vi "Recieve M1M3 State Event.vi"(8 "error in (no error)":errorcluster, 11 "M1M3 Support Events in":refnum<class "M1M3 Support Events.lvclass">) -> (0 "error out":errorcluster, 2 "M1M3 State":string, 3 "M1M3 Support Events out":refnum<class "M1M3 Support Events.lvclass">)   [LabVIEW 2016, in "M1M3 Support Events.lvclass"]
uses:
  M1M3 Support Events.lvclass
  M1M3 Support Events.lvclass/M1M3 Support Events.ctl
  Typedefs/StateTypes.ctl
  Typedefs/M1M3SupportEUI_TypeDefs.lvlib
  View/M1M3SupportEUI_Views.lvlib
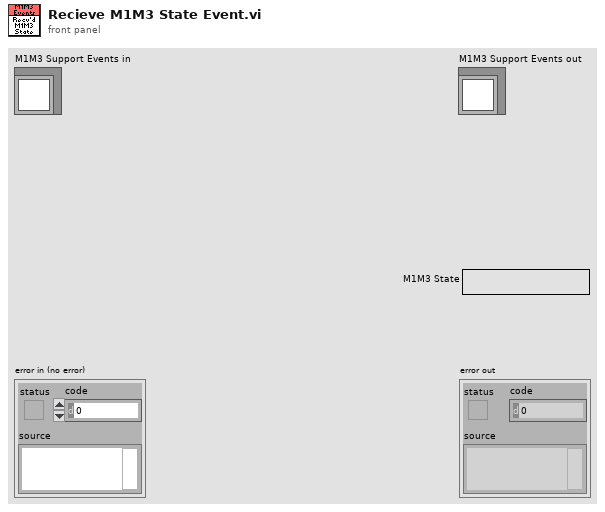
[diagram p1: front panel]
types:
  T1 = typedef "M1M3SupportEUI_TypeDefs.lvlib/M1M3 Support Events.ctl" = cluster{"M1M3 Support State":refnum<user-event>, "Inclinometer  Data":refnum<user-event>, "IMS Data":refnum<user-event>, "FA Status":refnum<user-event>, "SAL Connected":refnum<user-event>, "HP Data":refnum<user-event>, "HP Status":refnum<user-event>, "Accelerometer Data":refnum<user-event>, "FPGA Data":refnum<user-event>, "Inclinometer Data":refnum<user-event>, "MirrorForces Data":refnum<user-event>, "OuterLoop Data":refnum<user-event>, "ErrorCode Event":refnum<user-event>, "InterlockStatus Event":refnum<user-event>, "InterlockWarning Event":refnum<user-event>, "FA Data":refnum<user-event>, "HPMonitorStatus Event":refnum<user-event>, "Gyro Data":refnum<user-event>}
  T2 = typedef "M1M3SupportEUI_TypeDefs.lvlib/StateTypes.ctl" = u32
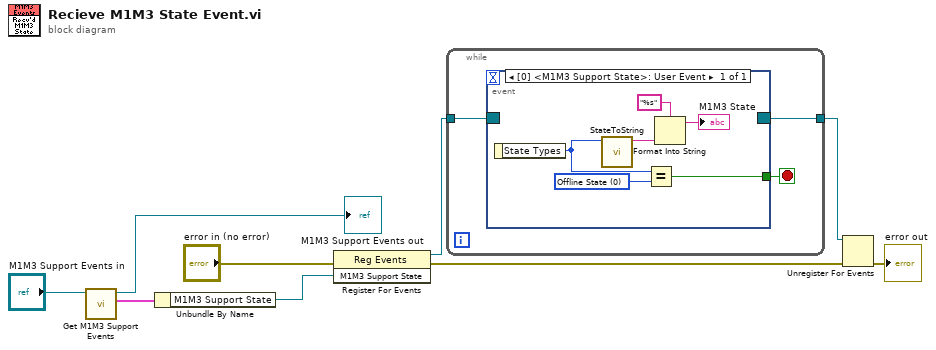
[diagram p0: block diagram]
diagram:
  n1 = call "Get M1M3 Support Events.vi"("M1M3 Support Events in"="M1M3 Support Events in") -> ("M1M3 Support Events"=w9:T1, "M1M3 Support Events out"=→"M1M3 Support Events out":refnum<class "M1M3 Support Events.lvclass">)  [unwired: 9 in]
  n2 = Unbundle By Name(w9) -> ("M1M3 Support State"=w6:refnum<user-event>)
  n3 = register-events(error in="error in (no error)", w6) -> (reference out=w5:refnum<event-registration>, error out=w2:errorcluster)  [unwired: 1 in]
  n4 = while {
    tunnel: w5 -> [w12]
    tunnel: [w10] -> w4
    stop <- w11 stop-if-true
    n5 = event shown="[0] <M1M3 Support State>: User Event" {
      selector: w12 -> [_]
      dyn-events: [_] -> w10
      timeout: _ -> [_]
      tunnel: [w15] -> w11
      event User Event {
        w16 = T2 0 items=["Offline State"=0, "Fault State"=4294967295, "Standby State"=16777216, "Disabled State"=33554432, "Enabled State"=50331648, "Parked State"=50331649, "Raising State"=50331650, "Active State"=50331651, "Lowering State"=50331652, "Engineering State"=50397184, "Parked Engineering State"=50397185, "Raising Engineering State"=50397186, "Active Engineering State"=50397187, "Lowering Engineering State"=50397188] ("y")
        n6 = event-data() -> ("State Types"=w14:T2)  [unwired: 1 in]
        n7 = call "StateToString.vi"("State Type Numeric"=w14) -> ("State Type String"=w13:string)  [unwired: 10 in]
        n8 = Equal?(x=w14, y=w16) -> (x = y?=w15:bool)
        n9 = Format Into String(format string="%s", w13) -> (resulting string=→"M1M3 State":string)  [unwired: 2 in, 1 out]
      }
    }
  }
  n10 = Unregister For Events(event registration refnum=w4, error in=w2) -> (error out=→"error out":errorcluster)
